vi "example_02_file.vi"() -> ()   [LabVIEW 2015, in "lv-dialog.lvlib"]
uses:
  lv-dialog.lvlib
panel:
  out "selected_path":path
  out "error out":errorcluster
  in  "start_path":path
  in  "title":string
  in  "filter":string="All files (*.*)|*.*"
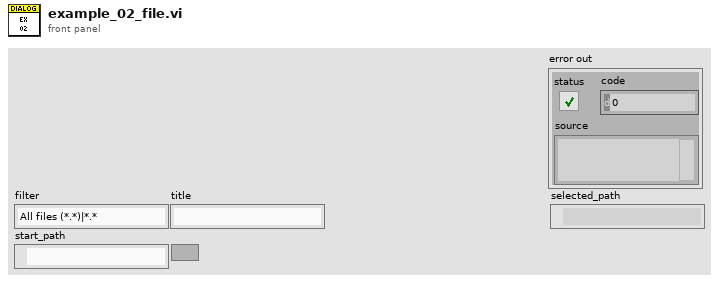
[diagram p1: front panel]
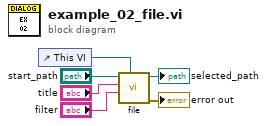
[diagram p0: block diagram]
diagram:
  n1 = control-ref of="This VI"() -> (w1:refnum<vi>)
  n2 = call "file.vi"("calling_vi"=w1, "filter"="filter", "title"="title", "start_path"="start_path") -> ("error out"=→"error out":errorcluster, "selected_path"=→"selected_path":path)  [unwired: 6 in]
